vi "GoalKickKeeperRoleVSS.vi"(7 "First call?":bool=TRUE, 8 "error in (no error)":errorcluster, 10 "Game in":refnum<class "Game.lvclass">, 11 "GoalKickKeeperRoleVSS in":refnum<class "GoalKickKeeperRoleVSS.lvclass">) -> (0 "error out":errorcluster, 1 "Robot out":refnum<class "Robot.lvclass">, 2 "Game out":refnum<class "Game.lvclass">, 3 "GoalKickKeeperRoleVSS out":refnum<class "GoalKickKeeperRoleVSS.lvclass">)   [LabVIEW 2023, in "GoalKickKeeperRoleVSS.lvclass"]
uses:
  GoalKickKeeperRoleVSS.lvclass
  Robot_class/Robot.lvclass
  Game_class/Game.lvclass
  Role_class/Role.lvclass/Role.ctl
  Role_class/Read Tacticbook.vi
  Role_class/Read tactic_index.vi
  Role_class/Write Tacticbook.vi
  Role_class/Write tactic_index.vi
  Role_class/Read RobotRef.vi
  Tacticbook_class/Tacticbook.lvclass
  DispBallTacticVSS_class/DispBallTacticVSS.lvclass
  DefendGoalTacticVSS_class/DefendGoalTacticVSS.lvclass
  PenaltyAttackTacticVSS_class/PenaltyAttackTacticVSS.lvclass
  DefendAreaTacticVSS_class/DefendAreaTacticVSS.lvclass
  AttackTacticVSS_class/AttackTacticVSS.lvclass
  HaltTactic_class/HaltTactic.lvclass
  GoAndKickTacticVSS_class/GoAndKickTacticVSS.lvclass
  GoalKickKeeperTacticVSS_class/GoalKickKeeperTacticVSS.lvclass
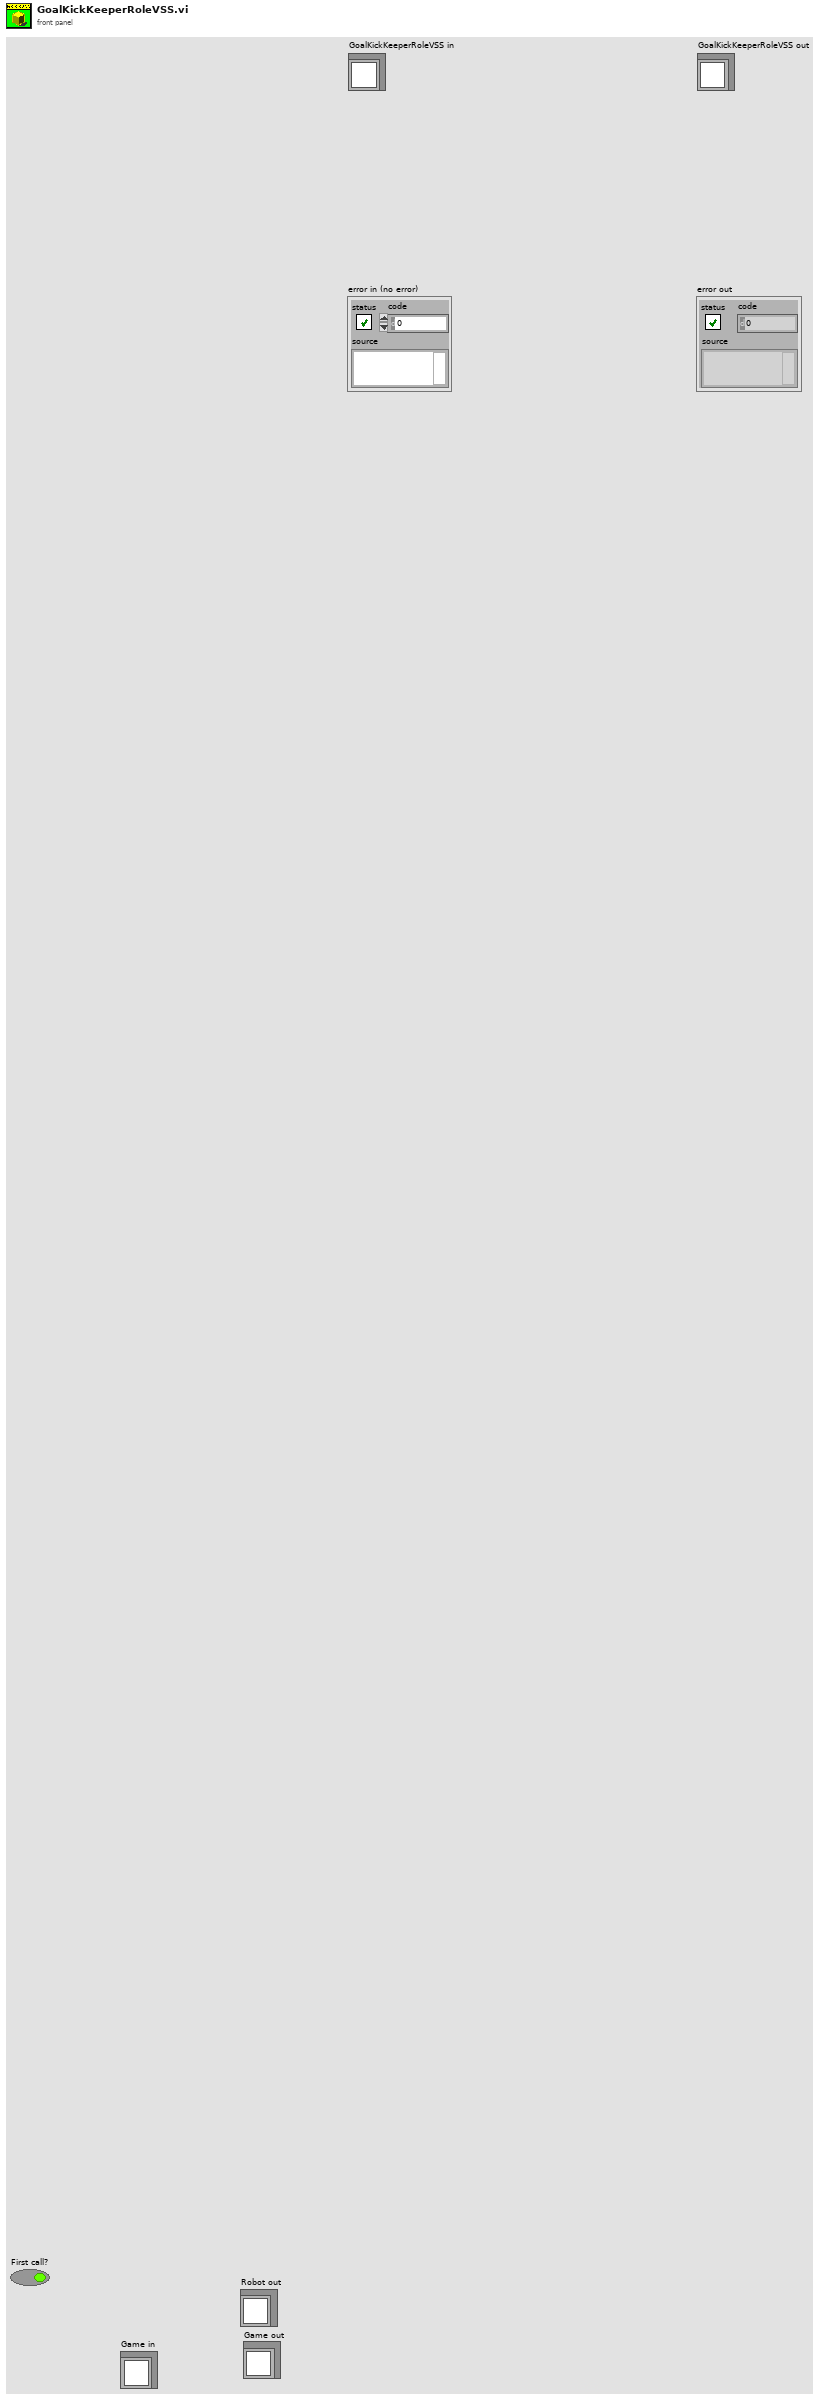
[diagram p1: front panel]
types:
  T1 = cluster{"DispBallTacticVSS":refnum<class "DispBallTacticVSS.lvclass">, "DefendGoalTacticVSS":refnum<class "DefendGoalTacticVSS.lvclass">, "PenaltyAttackTacticVSS":refnum<class "PenaltyAttackTacticVSS.lvclass">, "DefendAreaTacticVSS":refnum<class "DefendAreaTacticVSS.lvclass">, "AttackTacticVSS":refnum<class "AttackTacticVSS.lvclass">, "HaltTactic":refnum<class "HaltTactic.lvclass">, "GoAndKickTacticVSS":refnum<class "GoAndKickTacticVSS.lvclass">, "GoalKickKeeperTacticVSS":refnum<class "GoalKickKeeperTacticVSS.lvclass">}
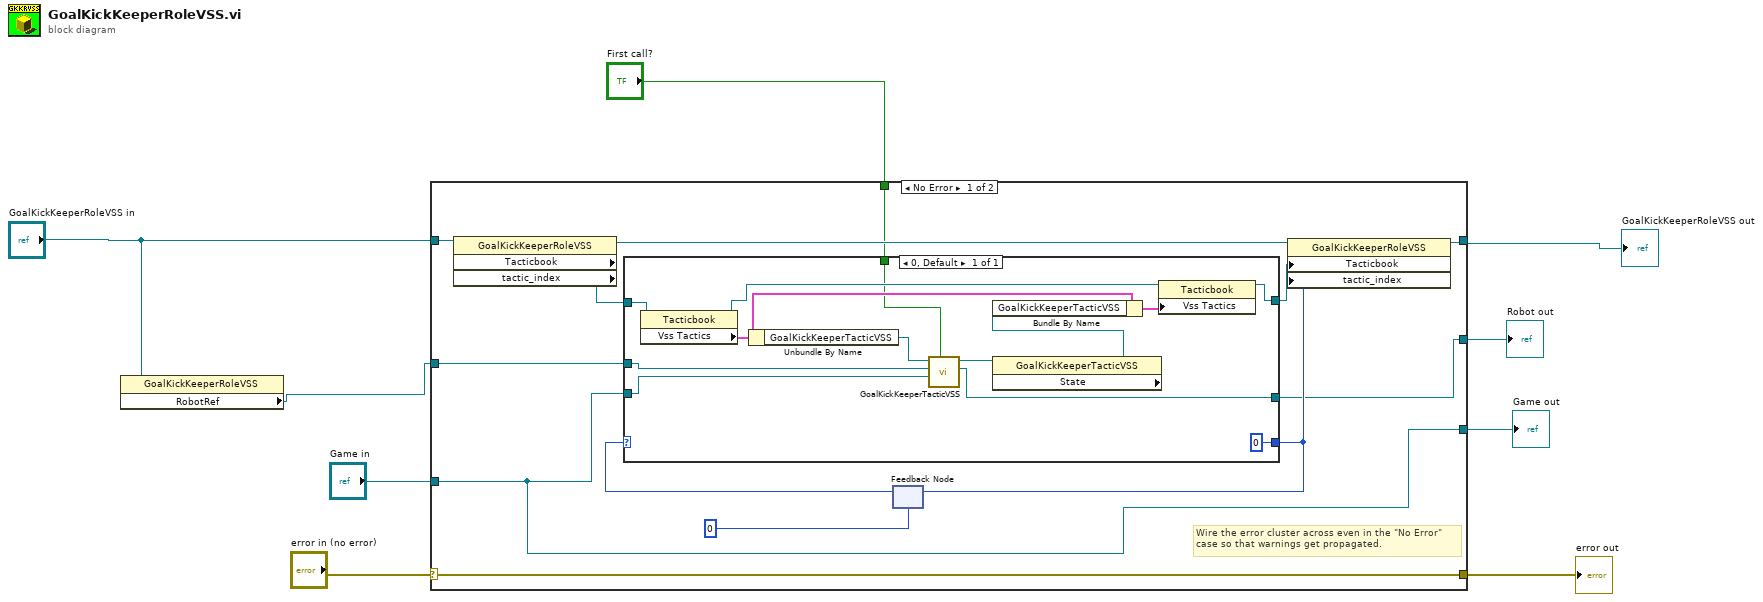
[diagram p0: block diagram]
diagram:
  n1 = property class="GoalKickKeeperRoleVSS"(reference="GoalKickKeeperRoleVSS in") -> ("RobotRef"=w6:refnum<class "Robot.lvclass">)  [unwired: 1 in, 2 out]
  n2 = case shown="No Error" "error in (no error)" {
    selector: "error in (no error)" -> [w22 w39]
    tunnel: [w22 w39] -> w3
    tunnel: [w20 w38] -> w4
    tunnel: "GoalKickKeeperRoleVSS in" -> [w21 w38]
    tunnel: w6 -> [w14 w37]
    tunnel: [w10 w37] -> w9
    tunnel: [w12 w36] -> w8
    tunnel: "Game in" -> [w12 w36]
    tunnel: "First call?" -> [w11 _]
    frame No Error {
      # "Wire the error cluster across even in the \"No Error\"\ncase so that warnings get propagated."
      n3 = property class="GoalKickKeeperRoleVSS" props=["Tacticbook", "tactic_index"](reference=w21) -> (reference out=w19:refnum<class "GoalKickKeeperRoleVSS.lvclass">, "Tacticbook"=w16:refnum<class "Tacticbook.lvclass">)  [unwired: 1 in, 2 out]
      n4 = feedback #1(0) -> (w17:i32)
      n5 = case shown="0, Default" w17 {
        tunnel: [0] -> w15
        tunnel: w16 -> [w35]
        tunnel: w14 -> [w26]
        tunnel: [w33] -> w13
        tunnel: w12 -> [w25]
        tunnel: w11 -> [w24]
        tunnel: [w23] -> w10
        frame 0, Default {
          n6 = property class="Tacticbook"(reference=w35) -> (reference out=w34:refnum<class "Tacticbook.lvclass">, "Vss Tactics"=w31:T1)  [unwired: 1 in, 1 out]
          n7 = Unbundle By Name(w31) -> ("GoalKickKeeperTacticVSS"=w27:refnum<class "GoalKickKeeperTacticVSS.lvclass">)
          n8 = call "GoalKickKeeperTacticVSS.vi"("First call?"=w24, "Game in"=w25, "Robot"=w26, "GoalKickKeeperTacticVSS in"=w27) -> ("Robot out"=w23:refnum<class "Robot.lvclass">, "GoalKickKeeperTacticVSS out"=w28:refnum<class "GoalKickKeeperTacticVSS.lvclass">)  [unwired: 4 in, 2 out]
          n9 = property class="GoalKickKeeperTacticVSS" props=["State"](reference=w28) -> (reference out=w29:refnum<class "GoalKickKeeperTacticVSS.lvclass">)  [unwired: 1 in, 2 out]
          n10 = Bundle By Name(cluster=w31, "GoalKickKeeperTacticVSS"=w29) -> (w30:T1)
          n11 = property class="Tacticbook"(reference=w34, "Vss Tactics"=w30) -> (reference out=w33:refnum<class "Tacticbook.lvclass">)  [unwired: 1 in, 1 out]
        }
      }
      n12 = feedback-in #1(w15) -> ()
      n13 = property class="GoalKickKeeperRoleVSS"(reference=w19, "Tacticbook"=w13, "tactic_index"=w15) -> (reference out=w20:refnum<class "GoalKickKeeperRoleVSS.lvclass">)  [unwired: 1 in, 1 out]
    }
    frame Error {
    }
  }
  "error out" <- w3
  "GoalKickKeeperRoleVSS out" <- w4
  "Robot out" <- w9
  "Game out" <- w8
